vi "Strafe_Correction.vi"(8 "error in":errorcluster) -> ()   [LabVIEW 2018]
panel:
  # ".035"
  # "0"
  # ".002"
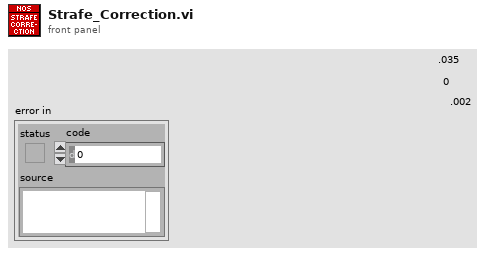
[diagram p1: front panel]
types:
  T1 = cluster{"proportional gain (Kc)":dbl, "integral time (Ti, min)":dbl, "derivative time (Td, min)":dbl}
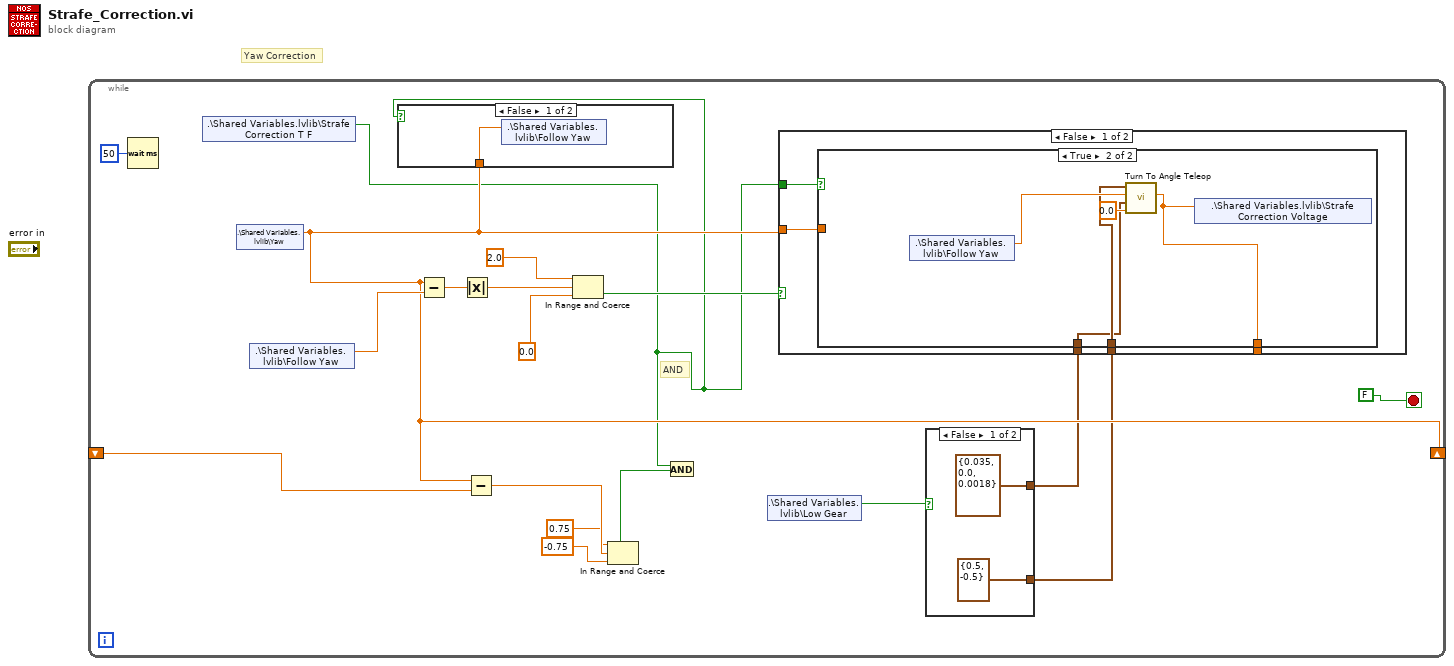
[diagram p0: block diagram]
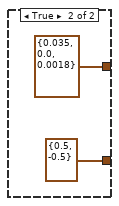
[diagram p2: hidden frame]
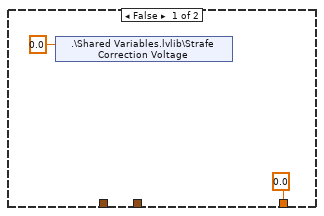
[diagram p4: hidden frame]
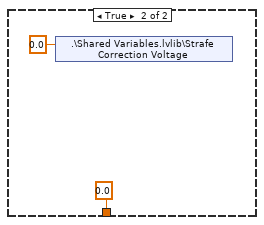
[diagram p5: hidden frame]
diagram:
  # "Yaw Correction"
  n1 = while {
    shift-right: [w10] -> _
    shift-left: _ -> [w9]
    stop <- FALSE stop-if-true
    # "AND"
    n2 = Wait (ms)(milliseconds to wait=u32 50) -> ()  [unwired: 1 out]
    n3 = shared-variable ".\\Shared Variables.lvlib\\Strafe Correction T F"() -> (w2:bool)  [unwired: 1 in, 1 out]
    n4 = shared-variable ".\\Shared Variables.lvlib\\Yaw"() -> (w10:dbl)  [unwired: 1 in, 1 out]
    n5 = shared-variable ".\\Shared Variables.lvlib\\Follow Yaw"() -> (w16:dbl)  [unwired: 1 in, 1 out]
    n6 = case shown="False" w2 {
      tunnel: w10 -> [w23 _]
      frame False {
        n7 = shared-variable ".\\Shared Variables.lvlib\\Follow Yaw"(w23) -> ()  [unwired: 1 in, 1 out]
      }
      frame True {
      }
    }
    n8 = Subtract(x=w10, y=w16) -> (x-y=w13:dbl)
    n9 = Absolute Value(x=w13) -> (abs(x)=w12:dbl)
    n10 = Subtract(x=w10, y=w9) -> (x-y=w8:dbl)
    n11 = In Range and Coerce(upper limit=2.0, x=w12, lower limit=0.0) -> (In Range?=w14:bool)  [unwired: 1 out]
    n12 = In Range and Coerce(upper limit=0.75, x=w8, lower limit=-0.75) -> (In Range?=w1:bool)  [unwired: 1 out]
    n13 = And(x=w2, y=w1) -> ()  [unwired: 1 out]
    n14 = shared-variable ".\\Shared Variables.lvlib\\Low Gear"() -> (w5:bool)  [unwired: 1 in, 1 out]
    n15 = case shown="False" w5 {
      tunnel: [cluster{"output high":dbl, "output low":dbl} {"output high"=0.5, "output low"=-0.5} ("output range") cluster{"output high":dbl, "output low":dbl} {"output high"=0.5, "output low"=-0.5} ("output range")] -> w4
      tunnel: [T1 {"proportional gain (Kc)"=0.035, "integral time (Ti, min)"=0.0, "derivative time (Td, min)"=0.0018} ("PID gains") T1 {"proportional gain (Kc)"=0.035, "integral time (Ti, min)"=0.0, "derivative time (Td, min)"=0.0018} ("PID gains")] -> w3
      frame False {
      }
      frame True {
      }
    }
    n16 = case shown="False" w14 {
      tunnel: w10 -> [w28 _]
      tunnel: w2 -> [w27 _]
      tunnel: w4 -> [w26 _]
      tunnel: w3 -> [w25 _]
      tunnel: [w24 0.0] -> _
      frame False {
        n17 = case shown="True" w27 {
          tunnel: w28 -> [_ _]
          tunnel: w26 -> [_ w32]
          tunnel: w25 -> [_ w31]
          tunnel: [0.0 w35] -> w24
          frame False {
            n18 = shared-variable ".\\Shared Variables.lvlib\\Strafe Correction Voltage"(0.0 ("Strafe Correction Voltage")) -> ()  [unwired: 1 in, 1 out]
          }
          frame True {
            n19 = shared-variable ".\\Shared Variables.lvlib\\Follow Yaw"() -> (w33:dbl)  [unwired: 1 in, 1 out]
            n20 = call "Turn To Angle Teleop.vi"("Z Axis"=0.0, "PID gains"=w31, "POV"=w33, "output range"=w32) -> ("Adjustment Voltage"=w35:dbl)  [unwired: 7 in]
            n21 = shared-variable ".\\Shared Variables.lvlib\\Strafe Correction Voltage"(w35) -> ()  [unwired: 1 in, 1 out]
          }
        }
      }
      frame True {
        n22 = shared-variable ".\\Shared Variables.lvlib\\Strafe Correction Voltage"(0.0 ("Strafe Correction Voltage")) -> ()  [unwired: 1 in, 1 out]
      }
    }
  }
